vi "Primary Density.vi"(10 "Pri Cold Temp":dbl, 11 "Pri Hot Temp":dbl) -> (1 "Primary Cold Density (kg/m^3)":dbl, 2 "Primary Hot Density (kg/m^3)":dbl, 3 "Primary Average Density (kg/m^3)":dbl)   [LabVIEW 2019]
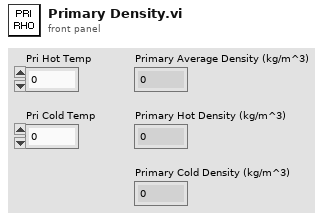
[diagram p1: front panel]
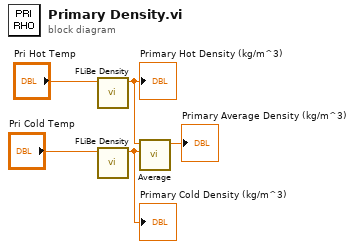
[diagram p0: block diagram]
diagram:
  n1 = call "FLiBe Density.vi"("Pri Temp (K)"="Pri Hot Temp") -> ("Primary Density (kg/m^3)"=w4:dbl)  [unwired: 10 in]
  "Primary Hot Density (kg/m^3)" <- w4
  n2 = call "FLiBe Density.vi"("Pri Temp (K)"="Pri Cold Temp") -> ("Primary Density (kg/m^3)"=w3:dbl)  [unwired: 10 in]
  "Primary Cold Density (kg/m^3)" <- w3
  n3 = call "Average.vi"("Number 2"=w3, "Number 1"=w4) -> ("Average"=→"Primary Average Density (kg/m^3)":dbl)  [unwired: 9 in]
